vi "BackpackCalculator.vi"(10 "Pot Value":dbl) -> (2 "Backpack Extension":dbl)   [LabVIEW 2014]
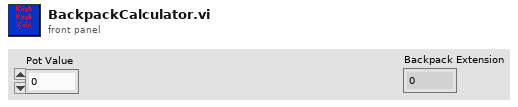
[diagram p1: front panel]
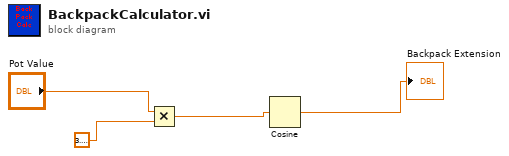
[diagram p0: block diagram]
diagram:
  n1 = Multiply(x="Pot Value", y=3.141592653589793) -> (x*y=w2:dbl)
  n2 = Cosine(x=w2) -> (cos(x)=→"Backpack Extension":dbl)
